vi "Init DAQs (In).vi"(8 "error in (no error)":errorcluster, 11 "Timing":T1={"Sampling Rate (Hz)"=1000.0, "Display Rate (Hz)"=100.0, "Sampling Mode"=2} {"Sampling Mode" items=["Finite Samples", "Continuous Samples", "Hardware Timed Single Point"]; "Sampling Rate (Hz)" format="%0.2f"}) -> (0 "error out":errorcluster, 2 "Channel Array":refnum<k21>[](array[refnum]))   [LabVIEW 2017]
uses:
  Controls/Timing Controls.ctl
  <vilib>/DAQmx/create/channels.llb/DAQmx Create Channel (AI-Voltage-Basic).vi
  <vilib>/DAQmx/configure/timing.llb/DAQmx Timing (Sample Clock).vi
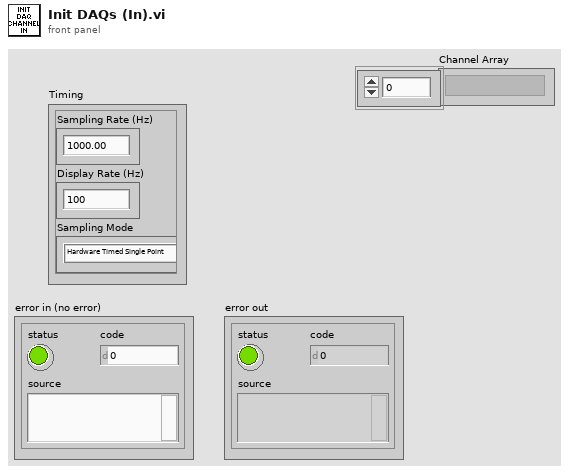
[diagram p1: front panel]
types:
  T1 = typedef "Timing Controls.ctl" = cluster{"Sampling Rate (Hz)":dbl, "Display Rate (Hz)":dbl, "Sampling Mode":i32}
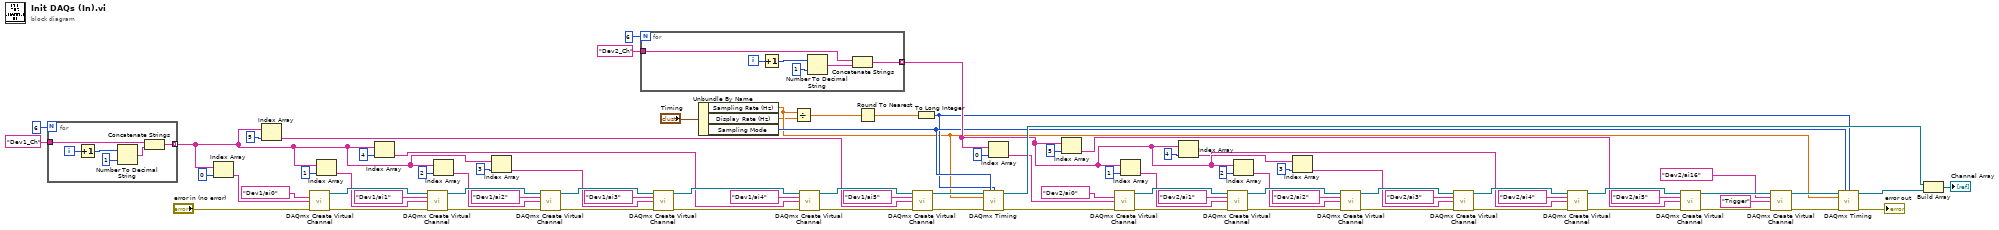
[diagram p0: block diagram]
diagram:
  n1 = for {
    N: 6 -> [_]
    tunnel: "Dev1_Ch" ("name to assign") -> [w85]
    tunnel: [w84] -> w11 mode=indexing
    i -> [w89]
    n2 = Increment(x=w89) -> (x+1=w87:i32)
    n3 = Number To Decimal String(number=w87, width (-)=i16 1) -> (decimal integer string=w86:string)
    n4 = Concatenate Strings(w85, w86) -> (w84:string)
  }
  n5 = Index Array(array=w11, index=0) -> (element=w17:string)
  n6 = Index Array(array=w11, index=5) -> (element=w6:string)
  n7 = call-poly <vilib>:"DAQmx Create Virtual Channel.vi"("physical channels"=tag "Dev1/ai0", "name to assign"=w17, "error in"="error in (no error)") -> ("task out"=w38:refnum<k21>, "error out"=w34:errorcluster)  [unwired: 11 in]
  n8 = Index Array(array=w11, index=1) -> (element=w10:string)
  n9 = Index Array(array=w11, index=4) -> (element=w7:string)
  n10 = call-poly <vilib>:"DAQmx Create Virtual Channel.vi"("task in"=w38, "physical channels"=tag "Dev1/ai1", "name to assign"=w10, "error in"=w34) -> ("task out"=w36:refnum<k21>, "error out"=w32:errorcluster)  [unwired: 10 in]
  n11 = Index Array(array=w11, index=2) -> (element=w9:string)
  n12 = Index Array(array=w11, index=3) -> (element=w8:string)
  n13 = call-poly <vilib>:"DAQmx Create Virtual Channel.vi"("task in"=w36, "physical channels"=tag "Dev1/ai2", "name to assign"=w9, "error in"=w32) -> ("task out"=w35:refnum<k21>, "error out"=w30:errorcluster)  [unwired: 10 in]
  n14 = for {
    N: 6 -> [_]
    tunnel: "Dev2_Ch" ("name to assign") -> [w91]
    tunnel: [w90] -> w48 mode=indexing
    i -> [w95]
    n15 = Increment(x=w95) -> (x+1=w93:i32)
    n16 = Number To Decimal String(number=w93, width (-)=i16 1) -> (decimal integer string=w92:string)
    n17 = Concatenate Strings(w91, w92) -> (w90:string)
  }
  n18 = call-poly <vilib>:"DAQmx Create Virtual Channel.vi"("task in"=w35, "physical channels"=tag "Dev1/ai3", "name to assign"=w8, "error in"=w30) -> ("task out"=w27:refnum<k21>, "error out"=w28:errorcluster)  [unwired: 10 in]
  n19 = Unbundle By Name("Timing") -> ("Sampling Rate (Hz)"=w2:dbl, "Display Rate (Hz)"=w1:dbl, "Sampling Mode"=w40:i32)
  n20 = Divide(x=w2, y=w1) -> (x/y=w4:dbl)
  n21 = call-poly <vilib>:"DAQmx Create Virtual Channel.vi"("task in"=w27, "physical channels"=tag "Dev1/ai4", "name to assign"=w7, "error in"=w28) -> ("task out"=w24:refnum<k21>, "error out"=w23:errorcluster)  [unwired: 10 in]
  n22 = Round To Nearest(number=w4) -> (nearest integer value=w5:dbl)
  n23 = call-poly <vilib>:"DAQmx Create Virtual Channel.vi"("task in"=w24, "physical channels"=tag "Dev1/ai5", "name to assign"=w6, "error in"=w23) -> ("task out"=w22:refnum<k21>, "error out"=w21:errorcluster)  [unwired: 10 in]
  n24 = To Long Integer(number=w5) -> (32bit integer=w3:i32)
  n25 = call-poly <vilib>:"DAQmx Timing.vi"("task/channels in"=w22, "sample mode"=w40, "samples per channel"=w3, "rate"=w2, "error in"=w21) -> ("task out"=w79:refnum<k21>, "error out"=w81:errorcluster)  [unwired: 9 in]
  n26 = Index Array(array=w48, index=0) -> (element=w49:string)
  n27 = Index Array(array=w48, index=5) -> (element=w43:string)
  n28 = call-poly <vilib>:"DAQmx Create Virtual Channel.vi"("physical channels"=tag "Dev2/ai0", "name to assign"=w49, "error in"=w81) -> ("task out"=w64:refnum<k21>, "error out"=w65:errorcluster)  [unwired: 11 in]
  n29 = Index Array(array=w48, index=1) -> (element=w47:string)
  n30 = Index Array(array=w48, index=4) -> (element=w44:string)
  n31 = call-poly <vilib>:"DAQmx Create Virtual Channel.vi"("task in"=w64, "physical channels"=tag "Dev2/ai1", "name to assign"=w47, "error in"=w65) -> ("task out"=w63:refnum<k21>, "error out"=w62:errorcluster)  [unwired: 10 in]
  n32 = Index Array(array=w48, index=2) -> (element=w46:string)
  n33 = Index Array(array=w48, index=3) -> (element=w45:string)
  n34 = call-poly <vilib>:"DAQmx Create Virtual Channel.vi"("task in"=w63, "physical channels"=tag "Dev2/ai2", "name to assign"=w46, "error in"=w62) -> ("task out"=w60:refnum<k21>, "error out"=w61:errorcluster)  [unwired: 10 in]
  n35 = call-poly <vilib>:"DAQmx Create Virtual Channel.vi"("task in"=w60, "physical channels"=tag "Dev2/ai3", "name to assign"=w45, "error in"=w61) -> ("task out"=w58:refnum<k21>, "error out"=w59:errorcluster)  [unwired: 10 in]
  n36 = call-poly <vilib>:"DAQmx Create Virtual Channel.vi"("task in"=w58, "physical channels"=tag "Dev2/ai4", "name to assign"=w44, "error in"=w59) -> ("task out"=w56:refnum<k21>, "error out"=w57:errorcluster)  [unwired: 10 in]
  n37 = call-poly <vilib>:"DAQmx Create Virtual Channel.vi"("task in"=w56, "physical channels"=tag "Dev2/ai5", "name to assign"=w43, "error in"=w57) -> ("task out"=w73:refnum<k21>, "error out"=w74:errorcluster)  [unwired: 10 in]
  n38 = call-poly <vilib>:"DAQmx Create Virtual Channel.vi"("task in"=w73, "physical channels"=tag "Dev2/ai16", "name to assign"="Trigger", "error in"=w74) -> ("task out"=w76:refnum<k21>, "error out"=w77:errorcluster)  [unwired: 10 in]
  n39 = call-poly <vilib>:"DAQmx Timing.vi"("task/channels in"=w76, "sample mode"=w40, "samples per channel"=w3, "rate"=w2, "error in"=w77) -> ("task out"=w42:refnum<k21>, "error out"=→"error out":errorcluster)  [unwired: 9 in]
  n40 = Build Array(w79, w42) -> (→"Channel Array":refnum<k21>[])
